vi "Add Port.vi"(7 "Highlight? (F)":bool, 8 "error in":errorcluster, 9 "redundant ?":bool, 10 "port Id":u32, 11 "ports ref":T1 format="%.0x") -> (0 "error out":errorcluster, 2 "port ref out":T1 format="%.0x", 3 "ports ref out":T1 format="%.0x")   [LabVIEW 2020, in "AIM ARINC 664 Scripting.lvlib"]
doc: "Add a port to the ports page with the specific port ID and redundancy."
uses:
  AIM ARINC 664 Scripting.lvlib
  <vilib>/NI VeriStand/Custom Device API/Custom Device Item Ref.ctl
  Import/_typedefs/port_setup.ctl
  Constants.vi
  <vilib>/NI VeriStand/Custom Device API/Custom Device API.lvlib
  Import/AIM ARINC 664 Import.lvlib
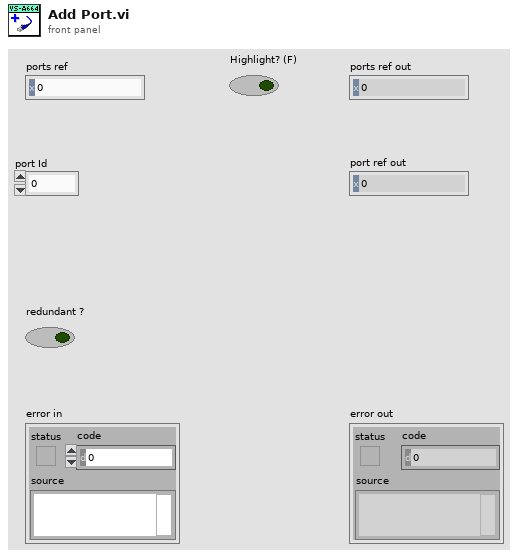
[diagram p1: front panel]
types:
  T1 = typedef "Custom Device API.lvlib/Custom Device Item Ref.ctl" = u64
  T2 = typedef "AIM ARINC 664 Import.lvlib/port_setup.ctl" = cluster{"port Id":u32, "redundant":bool}
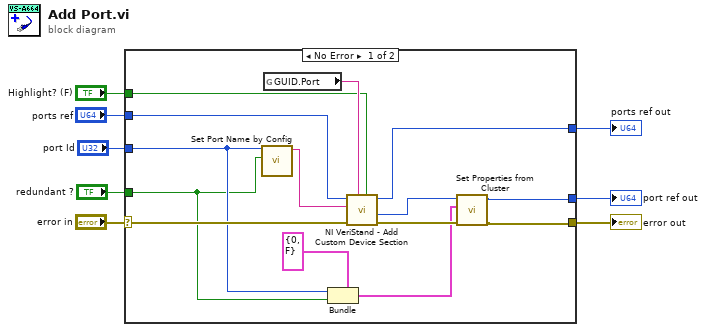
[diagram p0: block diagram]
diagram:
  n1 = case shown="No Error" "error in" {
    selector: "error in" -> [w19 w24]
    tunnel: "Highlight? (F)" -> [w21 _]
    tunnel: "ports ref" -> [w20 w23]
    tunnel: [w14 w24] -> w6
    tunnel: [w13 _] -> w5
    tunnel: [w18 w23] -> w3
    tunnel: "redundant ?" -> [w11 _]
    tunnel: "port Id" -> [w12 _]
    frame No Error {
      n2 = call "Set Port Name by Config.vi"("Redundant?"=w11, "port id"=w12) -> ("Port name out"=w17:string)  [unwired: 9 in]
      n3 = global read "Constants.vi" "GUID.Port"() -> (w22:string)
      n4 = Bundle(cluster=T2 {"port Id"=0, "redundant"=FALSE} ("portSetup"), "port Id"=w12, "redundant"=w11) -> (w10:T2)
      n5 = call <vilib>:"NI VeriStand - Add Custom Device Section.vi"("Highlight? (F)"=w21, "GUID (Default Section)"=w22, "error in (no error)"=w19, "Section Name"=w17, "Parent Ref in"=w20) -> ("error out"=w16:errorcluster, "Section Ptr"=w15:T1, "Parent Ref out"=w18:T1)  [unwired: 3 in, 1 out]
      n6 = call "Set Properties from Cluster.vi"("error in"=w16, "Variant Cluster"=w10, "item ref in"=w15) -> ("error out"=w14:errorcluster, "item ref out"=w13:T1)  [unwired: 7 in]
    }
    frame Error {
    }
  }
  "error out" <- w6
  "port ref out" <- w5
  "ports ref out" <- w3
